vi "Find Circle Center.vi"(8 "error in (no error)":errorcluster, 10 "X":dbl[](array[numeric]), 11 "Y":cluster{"Best Polynomial Fit":dbl[]}[](array[cluster])) -> (0 "error out":errorcluster, 2 "Y":dbl, 3 "X":dbl)   [LabVIEW 2009]
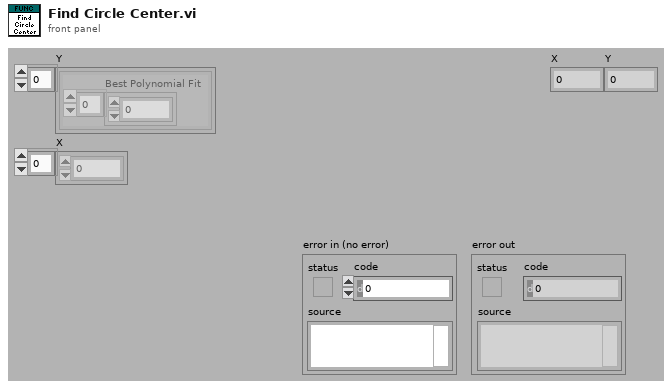
[diagram p1: front panel]
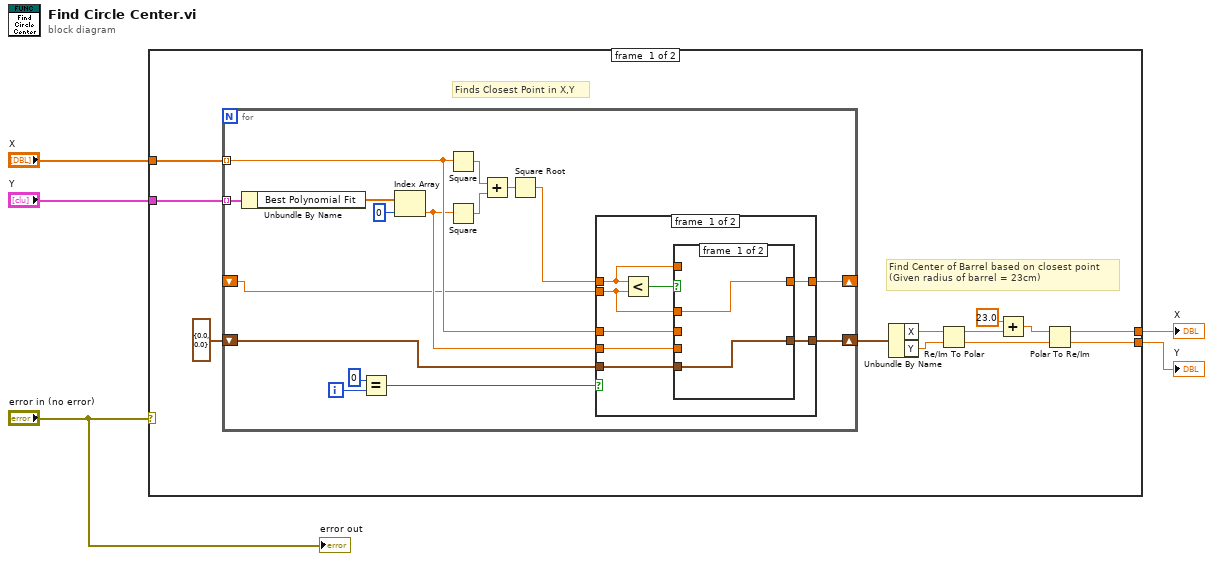
[diagram p0: block diagram]
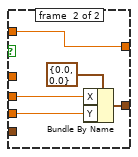
[diagram p2: hidden frame]
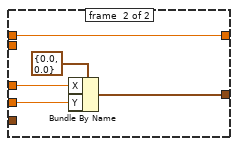
[diagram p3: hidden frame]
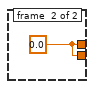
[diagram p4: hidden frame]
diagram:
  n1 = case shown="No Error" "error in (no error)" {
    tunnel: "Y" -> [w17 _]
    tunnel: "X" -> [w16 _]
    tunnel: [w7 w54] -> w3
    tunnel: [w6 w54] -> w2
    frame #0 {
      # "Find Center of Barrel based on closest point\n(Given radius of barrel = 23cm)"
      # "Finds Closest Point in X,Y"
      n2 = for {
        tunnel: w17 -> [w30] mode=indexing
        tunnel: w16 -> [w23] mode=indexing
        shift-right: [w24] -> _
        shift-left: _ -> [w20]
        shift-right: [w21] -> w10
        shift-left: cluster{"X":dbl, "Y":dbl} {"X"=0.0, "Y"=0.0} ("Cluster") -> [w19]
        i -> [w28]
        n3 = Unbundle By Name(w30) -> ("Best Polynomial Fit"=w18:dbl[])
        n4 = Equal?(x=0, y=w28) -> (x = y?=w26:bool)
        n5 = Index Array(array=w18, index=0) -> (element=w22:dbl)
        n6 = Square(x=w23) -> (x^2=w31:dbl)
        n7 = Square(x=w22) -> (x^2=w32:dbl)
        n8 = Add(x=w31, y=w32) -> (x+y=w33:dbl)
        n9 = Square Root(x=w33) -> (sqrt(x)=w25:dbl)
        n10 = case shown="False" w26 {
          tunnel: w25 -> [w37 w53]
          tunnel: [w36 w53] -> w24
          tunnel: w23 -> [w40 w51]
          tunnel: w22 -> [w39 w50]
          tunnel: [w38 w49] -> w21
          tunnel: w20 -> [w34 _]
          tunnel: w19 -> [w35 _]
          frame #0 {
            n11 = Less?(x=w37, y=w34) -> (x < y?=w41:bool)
            n12 = case shown="True" w41 {
              tunnel: w40 -> [_ w47]
              tunnel: w39 -> [_ w46]
              tunnel: [w43 w45] -> w38
              tunnel: w37 -> [_ w44]
              tunnel: [w42 w44] -> w36
              tunnel: w35 -> [w43 _]
              tunnel: w34 -> [w42 _]
              frame #0 {
              }
              frame #1 {
                n13 = Bundle By Name(cluster=cluster{"X":dbl, "Y":dbl} {"X"=0.0, "Y"=0.0} ("Cluster"), "X"=w47, "Y"=w46) -> (w45:cluster{"X":dbl, "Y":dbl})
              }
            }
          }
          frame #1 {
            n14 = Bundle By Name(cluster=cluster{"X":dbl, "Y":dbl} {"X"=0.0, "Y"=0.0} ("Cluster"), "X"=w51, "Y"=w50) -> (w49:cluster{"X":dbl, "Y":dbl})
          }
        }
      }
      n15 = Unbundle By Name(w10) -> ("X"=w9:dbl, "Y"=w8:dbl)
      n16 = Re/Im To Polar(2:w8, 3:w9) -> (0:w11:dbl, 1:w14:dbl)
      n17 = Add(x=23.0, y=w14) -> (x+y=w12:dbl)
      n18 = Polar To Re/Im(2:w11, 3:w12) -> (0:w6:dbl, 1:w7:dbl)
    }
    frame #1 {
      w54 = 0.0
    }
  }
  "X" <- w3
  "Y" <- w2
  "error out" <- "error in (no error)"
